vi "CSM - Status Change Event.vi"(8 "Error In":errorcluster caption="error in (no error)", 9 "Wait (5000ms)":i32=5000, 11 "CSM Module":string) -> (0 "error out":errorcluster, 1 "Waited (ms)":u32, 3 "Status Change Event":refnum<user-event>)   [LabVIEW 2017, in "Communicable State Machine.lvlib"]
doc: "### CSM - Status Change Event.vi\n\nGet the CSM status change event handle.\n\n-- <b>Controls</b> --\n- <b>CSM Module</b>: CSM module name\n\n-- <b>Indicators</b> --\n- <b>Status Change Event</b>: CSM status change event handle"
uses:
  _Support/Typedef/_CSM Status Change Event Data.ctl
  _Support/CSMQ/_CSMOFGVOPER.ctl
  Communicable State Machine.lvlib
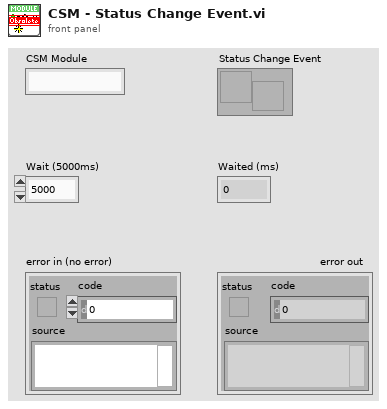
[diagram p1: front panel]
types:
  T1 = typedef "Communicable State Machine.lvlib/_CSMOFGVOPER.ctl" = enum16{"Create If not Exist", "Get By Name", "List", "Check If Name Exists", "Release", "Module Status", "Create Status Event Handler", "Destroy Status Event Handler", "Clear Invalid Objs"}
  T2 = typedef "Communicable State Machine.lvlib/_CSMObj.ctl" = cluster{"info":T3, "Refs":T5}
  T3 = typedef "Communicable State Machine.lvlib/_CSMObj-Info.ctl" = cluster{"Module Name":string, "Requested Name":string, "Group Name":string, "Mode":T4, "Allowed Messages":string[]}
  T4 = typedef "Communicable State Machine.lvlib/_CSM_MODE.ctl" = enum16{"Not Exist", "Stand Alone", "CSM", "Worker", "Worker Agent", "Chain Node", "Chain"}
  T5 = typedef "Communicable State Machine.lvlib/_CSMObj-Refs.ctl" = cluster{"WatchDogQ":refnum<queue>, "CSMDataDVR":refnum<data-value>, "Queue":T6, "GroupDataDVR":refnum<data-value>, "TagMap":refnum<data-value>, "ExitEvent":refnum<user-event>, "NewStateEvent":refnum<user-event>, "StatusChangeEvent":refnum<user-event>}
  T6 = typedef "Communicable State Machine.lvlib/Priority Queue.ctl" = cluster{"HPriorityQ":refnum<queue>, "LowPriorityQ":refnum<queue>}
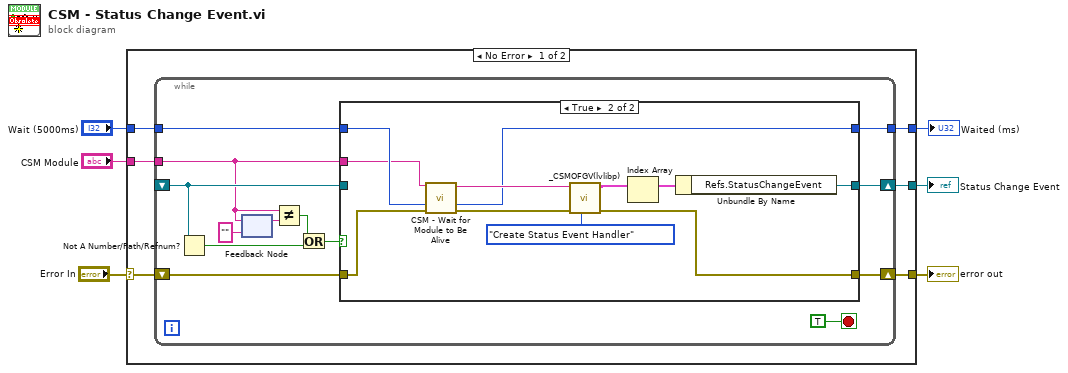
[diagram p0: block diagram]
diagram:
  n1 = case shown="No Error" "Error In" {
    selector: "Error In" -> [w11 w39]
    tunnel: [w12 _] -> w4
    tunnel: [w10 w39] -> w5
    tunnel: "CSM Module" -> [w9 _]
    tunnel: "Wait (5000ms)" -> [w8 _]
    tunnel: [w7 _] -> w1
    frame No Error {
      n2 = while {
        shift-right: [w23] -> w10
        shift-left: w11 -> [w24]
        shift-right: [w25] -> w12
        shift-left: _ -> [w21]
        tunnel: w9 -> [w19]
        tunnel: w8 -> [w14]
        tunnel: [w13] -> w7
        stop <- TRUE stop-if-true
        n3 = Not A Number/Path/Refnum?(number/path/refnum=w21) -> (NaN/Path/Refnum?=w17:bool)
        n4 = feedback-in #1(w19) -> ()
        n5 = feedback #1("" ("CSM Module")) -> (w18:string)
        n6 = Not Equal?(x=w19, y=w18) -> (x != y?=w16:bool)
        n7 = Or(x=w16, y=w17) -> (x .or. y?=w20:bool)
        n8 = case shown="True" w20 {
          tunnel: [w27 w34] -> w25
          tunnel: w24 -> [w26 w33]
          tunnel: [w26 w37] -> w23
          tunnel: w21 -> [w27 _]
          tunnel: w19 -> [_ w29]
          tunnel: w14 -> [_ w30]
          tunnel: [_ w28] -> w13
          frame False {
          }
          frame True {
            n9 = call "CSM - Wait for Module to Be Alive.vi"("CSM Name"=w29, "Wait (5000 ms)"=w30, "error in (no error)"=w33) -> ("CSM Name (Dup)"=w31:string, "Waited (ms)"=w28:u32, "error out"=w32:errorcluster)  [unwired: 10 in]
            n10 = call "_CSMOFGV(lvlibp).vi"("Operation"=_CSMOFGVOPER."Create Status Event Handler", "Error In"=w32, "Name (\"\" to Use UUID) In"=w31) -> ("error out"=w37:errorcluster, "Array"=w36:T2[])  [unwired: 6 in, 1 out]
            n11 = Index Array(array=w36) -> (element=w35:T2)  [unwired: 1 in]
            n12 = Unbundle By Name(w35) -> ("Refs.StatusChangeEvent"=w34:refnum<user-event>)
          }
        }
      }
    }
    frame Error {
    }
  }
  "error out" <- w5
  "Status Change Event" <- w4
  "Waited (ms)" <- w1
